vi "Main Page - Inline.vi"(8 "error in":errorcluster, 11 "Node Ptr":T1 format="%.0x") -> (0 "error out":errorcluster)   [LabVIEW 2026]
uses:
  <vilib>/NI VeriStand/Custom Device API/Custom Device Item Ref.ctl
  C:/Program Files/National Instruments/VeriStand 2026/NationalInstruments.VeriStand.Controls.dll
  Program Files/National Instruments/VeriStand 2026/NationalInstruments.VeriStand.Controls.dll
  <vilib>/NI VeriStand/Custom Device API/Custom Device API.lvlib
  Template System Explorer.lvlib
panel:
  in  "PagePropertyEditor":refnum<k24>(container)
  out "Version":string
  in  "Browser":refnum<k7>(container)
  in  "General Header":cluster{"Section Name":string}={"Section Name"="General Custom Device Settings"}
  in  "Description":string
  in  "Name":string
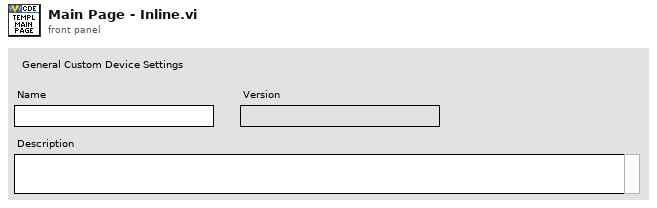
[diagram p1: front panel]
types:
  T1 = typedef "Custom Device API.lvlib/Custom Device Item Ref.ctl" = u64
  T2 = typedef "Custom Device API.lvlib/Custom Device Item Info.ctl" = cluster{"Name":string, "Is Channel":bool, "GUID":string, "Is Waveform":bool}
  T3 = typedef "Custom Device API.lvlib/Custom Device Commands.ctl" = enum16{"Default", "Item renamed", "Shutdown", "Dynamic button pressed"}
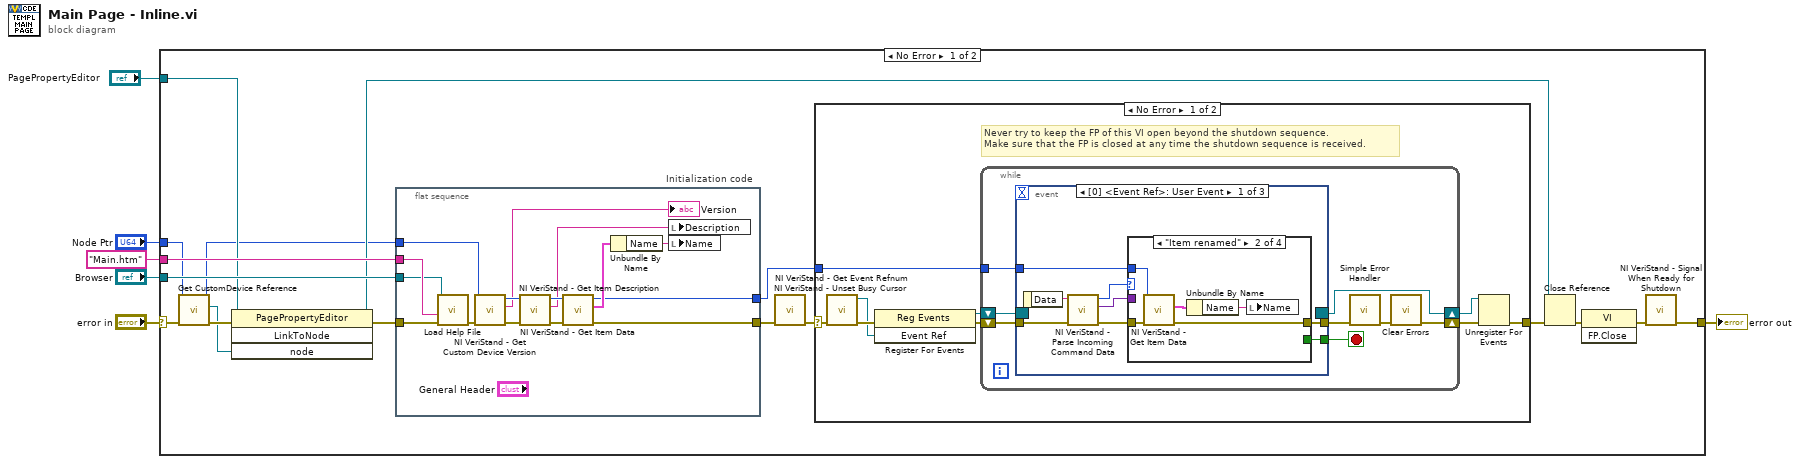
[diagram p0: block diagram]
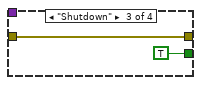
[diagram p3: hidden frame]
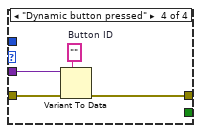
[diagram p4: hidden frame]
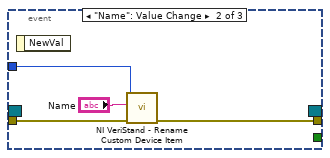
[diagram p5: hidden frame]
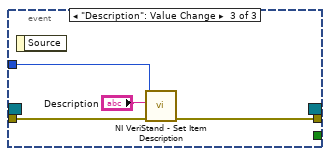
[diagram p6: hidden frame]
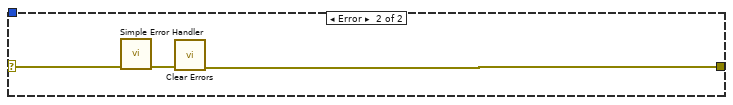
[diagram p7: hidden frame]
diagram:
  n1 = case shown="No Error" "error in" {
    selector: "error in" -> [w16 w87]
    tunnel: [w23 w87] -> w2
    tunnel: "Node Ptr" -> [w7 _]
    tunnel: "Browser" -> [w22 _]
    tunnel: "Main.htm" ("HTML File") -> [w21 _]
    tunnel: "PagePropertyEditor" -> [w9 _]
    frame No Error {
      n2 = call "Get CustomDevice Reference.vi"("error in"=w16, "Node Ptr"=w7) -> ("error out"=w12:errorcluster, "Custom Device"=w11:refnum<k24>, "Node Ptr"=w8:T1)  [unwired: 7 in]
      n3 = invoke class="PagePropertyEditor" method="LinkToNode"(reference=w9, error in=w12, "node"=w11) -> (reference out=w10:refnum<k24>, error out=w15:errorcluster)  [unwired: 1 in, 2 out]
      n4 = flat-sequence "Initialization code" {
        tunnel: w15 -> [w36]
        tunnel: w8 -> [w32]
        tunnel: [w24] -> w17
        tunnel: [w25] -> w18
        tunnel: w22 -> [w26]
        tunnel: w21 -> [w27]
        frame #0 {
          n5 = call "Load Help File.vi"("error in"=w36, "HTML File to Load"=w27, "Browser"=w26) -> ("error out"=w35:errorcluster)  [unwired: 8 in]
          n6 = call <vilib>:"NI VeriStand - Get Custom Device Version.vi"("error in (no error)"=w35, "Device Ref in"=w32) -> ("error out"=w37:errorcluster, "Value"=→"Version":string, "Device Ref out"=w31:T1)  [unwired: 7 in]
          n7 = call <vilib>:"NI VeriStand - Get Item Description.vi"("error in (no error)"=w37, "Item Ref in"=w31) -> ("error out"=w38:errorcluster, "Description"=w28:string, "Item Ref out"=w34:T1)  [unwired: 7 out]
          n8 = call <vilib>:"NI VeriStand - Get Item Data.vi"("error in (no error)"=w38, "Item Ref in"=w34) -> ("error out"=w24:errorcluster, "Item Info"=w33:T2, "Item Ref out"=w25:T1)  [unwired: 7 out]
          n9 = Unbundle By Name(w33) -> ("Name"=w29:string)
          n10 = local write "Description"(w28) -> ()
          n11 = local write "Name"(w29) -> ()
        }
      }
      n12 = call <vilib>:"NI VeriStand - Unset Busy Cursor.vi"("error in (no error)"=w17) -> ("error out"=w19:errorcluster)  [unwired: 10 out]
      n13 = case shown="No Error" w19 {
        selector: w19 -> [w43 w86]
        tunnel: [w45 w84] -> w14
        tunnel: w18 -> [w39 _]
        frame No Error {
          # "Never try to keep the FP of this VI open beyond the shutdown sequence.\nMake sure that the FP is closed at any time the shutdown sequence is received."
          n14 = call <vilib>:"NI VeriStand - Get Event Refnum.vi"("error in (no error)"=w43) -> ("error out"=w47:errorcluster, "Event Ref"=w41:refnum<user-event>)  [unwired: 9 out]
          n15 = register-events(error in=w47, w41) -> (reference out=w40:refnum<event-registration>, error out=w44:errorcluster)  [unwired: 1 in]
          n16 = while {
            tunnel: w39 -> [w48]
            shift-right: [w52] -> w46
            shift-left: w44 -> [w55]
            shift-right: [w51] -> w42
            shift-left: w40 -> [w50]
            stop <- w49 stop-if-true
            n17 = event shown="[0] <Event Ref>: User Event" {
              selector: w50 -> [_ _ _]
              dyn-events: [_ _ _] -> w51
              timeout: _ -> [_ _ _]
              tunnel: w55 -> [w63 w79 w83]
              tunnel: [w58 _ _] -> w49
              tunnel: [w61 w78 w82] -> w54
              tunnel: w48 -> [w57 w77 w81]
              event User Event {
                n18 = event-data() -> ("Data"=w60:string)  [unwired: 1 out]
                n19 = call <vilib>:"NI VeriStand - Parse Incoming Command Data.vi"("error in (no error)"=w63, "Incoming data"=w60) -> ("error out"=w62:errorcluster, "Outgoing data"=w56:variant, "Action"=w59:T3)  [unwired: 7 out]
                n20 = case shown="\"Item renamed\"" w59 {
                  tunnel: w62 -> [w64 w69 w71 w75]
                  tunnel: [_ _ TRUE _] -> w58
                  tunnel: [w64 w68 w71 w74] -> w61
                  tunnel: w57 -> [_ w67 _ _]
                  tunnel: w56 -> [_ _ _ w73]
                  frame "Default", Default {
                  }
                  frame "Item renamed" {
                    n21 = call <vilib>:"NI VeriStand - Get Item Data.vi"("error in (no error)"=w69, "Item Ref in"=w67) -> ("error out"=w68:errorcluster, "Item Info"=w66:T2)  [unwired: 8 out]
                    n22 = Unbundle By Name(w66) -> ("Name"=w65:string)
                    n23 = local write "Name"(w65) -> ()
                  }
                  frame "Shutdown" {
                  }
                  frame "Dynamic button pressed" {
                    w72 = ""  # Button ID
                    n24 = Variant To Data(error in=w75, type=w72, Variant=w73) -> (error out=w74:errorcluster)  [unwired: 1 out]
                  }
                }
              }
              event "Name": Value Change {
                n25 = event-data() -> ()  [unwired: 2 out]
                n26 = call <vilib>:"NI VeriStand - Rename Custom Device Item.vi"("error in (no error)"=w79, "New Name"="Name", "Item Ref in"=w77) -> ("error out"=w78:errorcluster)  [unwired: 1 in, 7 out]
              }
              event "Description": Value Change {
                n27 = event-data() -> ()  [unwired: 2 out]
                n28 = call <vilib>:"NI VeriStand - Set Item Description.vi"("error in (no error)"=w83, "Description"="Description", "Item Ref in"=w81) -> ("error out"=w82:errorcluster)  [unwired: 8 out]
              }
            }
            n29 = call <vilib>:"Simple Error Handler.vi"("error in (no error)"=w54) -> ("error out"=w53:errorcluster)  [unwired: 1 in, 7 out]
            n30 = call <vilib>:"Clear Errors.vi"("error in (no error)"=w53) -> ("error out"=w52:errorcluster)  [unwired: 1 in, 5 out]
          }
          n31 = Unregister For Events(event registration refnum=w42, error in=w46) -> (error out=w45:errorcluster)
        }
        frame Error {
          n32 = call <vilib>:"Simple Error Handler.vi"("error in (no error)"=w86) -> ("error out"=w85:errorcluster)  [unwired: 1 in, 7 out]
          n33 = call <vilib>:"Clear Errors.vi"("error in (no error)"=w85) -> ("error out"=w84:errorcluster)  [unwired: 1 in, 5 out]
        }
      }
      n34 = Close Reference(reference=w10, error in (no error)=w14) -> (error out=w13:errorcluster)
      n35 = invoke class="VI" method="FP.Close"(error in=w13) -> (error out=w20:errorcluster)  [unwired: 2 in, 2 out]
      n36 = call <vilib>:"NI VeriStand - Signal When Ready for Shutdown.vi"("error in (no error)"=w20) -> ("error out"=w23:errorcluster)  [unwired: 10 out]
    }
    frame Error {
    }
  }
  "error out" <- w2
